vi "4AnInsADS1115.vi"() -> ()   [LabVIEW 2024]
uses:
  Controls/ConfigData.ctl
  Controls/ADS1115Mode.ctl
  Controls/ADS1115Mux.ctl
  Controls/ADS1115DataRate.ctl
  Controls/ADS1115PGA.ctl
  Driver/CTIPicoVISA.lvlib
panel:
  in  "Numeric":u16
  out "Data 2":string
  out "string":string
  out "Data":string
  in  "Configure ADS1115":T1={"Mode"=enum."Single-Shot", "MUX"=enum."Single AI3 - GND", "Data Rate"=enum."8 SPS", "PGA"=enum."FS = ±6.144V"}
  out "Waveform Chart":dbl(graph)
  out "loop":i32
  out "Identity":T6
  in  "Grove Connector":enum16{"I2C0", "I2C1"}(ring)
  in  "stop":bool
  in  "VISA resource name in":refnum<visa-resource-name>="COM14"
  out "error out":errorcluster
  # "https://wiki.seeedstudio.com/Grove-16-bit-ADC-ADS1115/"
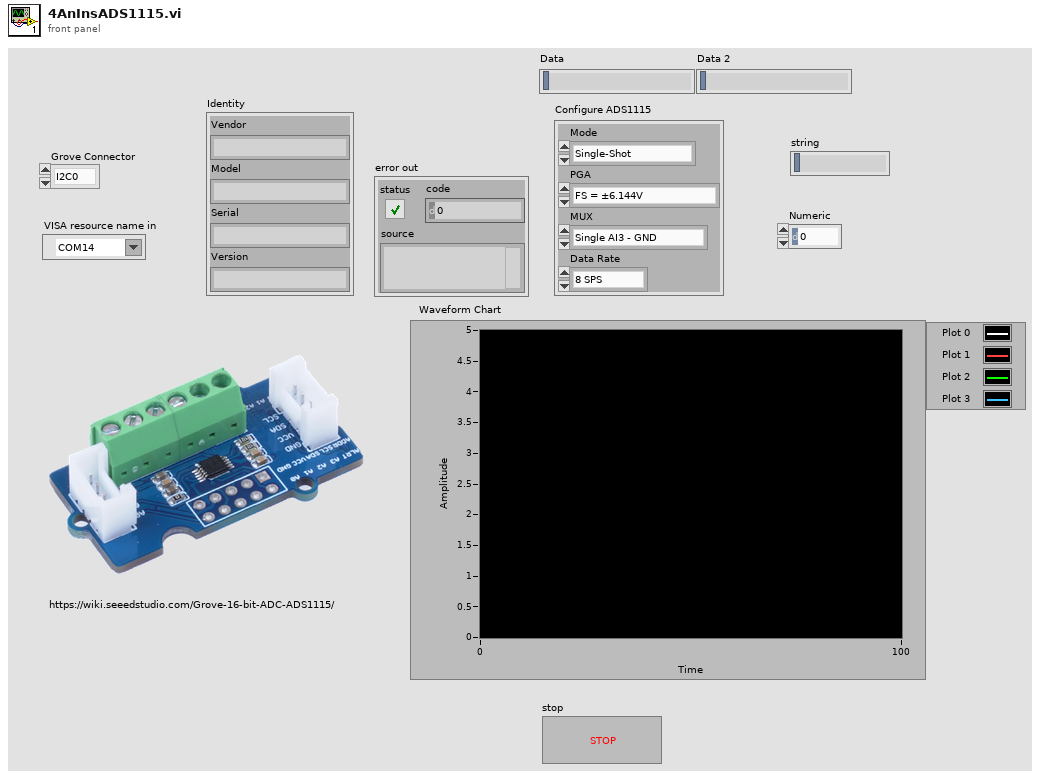
[diagram p1: front panel]
types:
  T1 = typedef "ConfigData.ctl" = cluster{"Mode":T2, "MUX":T3, "Data Rate":T4, "PGA":T5}
  T2 = typedef "ADS1115Mode.ctl" = enum16{"Continuous", "Single-Shot"}
  T3 = typedef "ADS1115Mux.ctl" = enum16{"Single AI0 - GND", "Single AI1 - GND", "Single AI2 - GND", "Single AI3 - GND"}
  T4 = typedef "ADS1115DataRate.ctl" = enum16{"8 SPS", "16 SPS", "32 SPS", "64 SPS", "128 SPS", "250 SPS", "475 SPS", "860 SPS"}
  T5 = typedef "ADS1115PGA.ctl" = enum16{"FS = ±6.144V", "FS = ±4.096V", "FS = ±2.048V", "FS = ±1.024V", "FS = ±0.512V", "FS = ±0.256V"}
  T6 = cluster{"Vendor":string, "Model":string, "Serial":string, "Version":string}
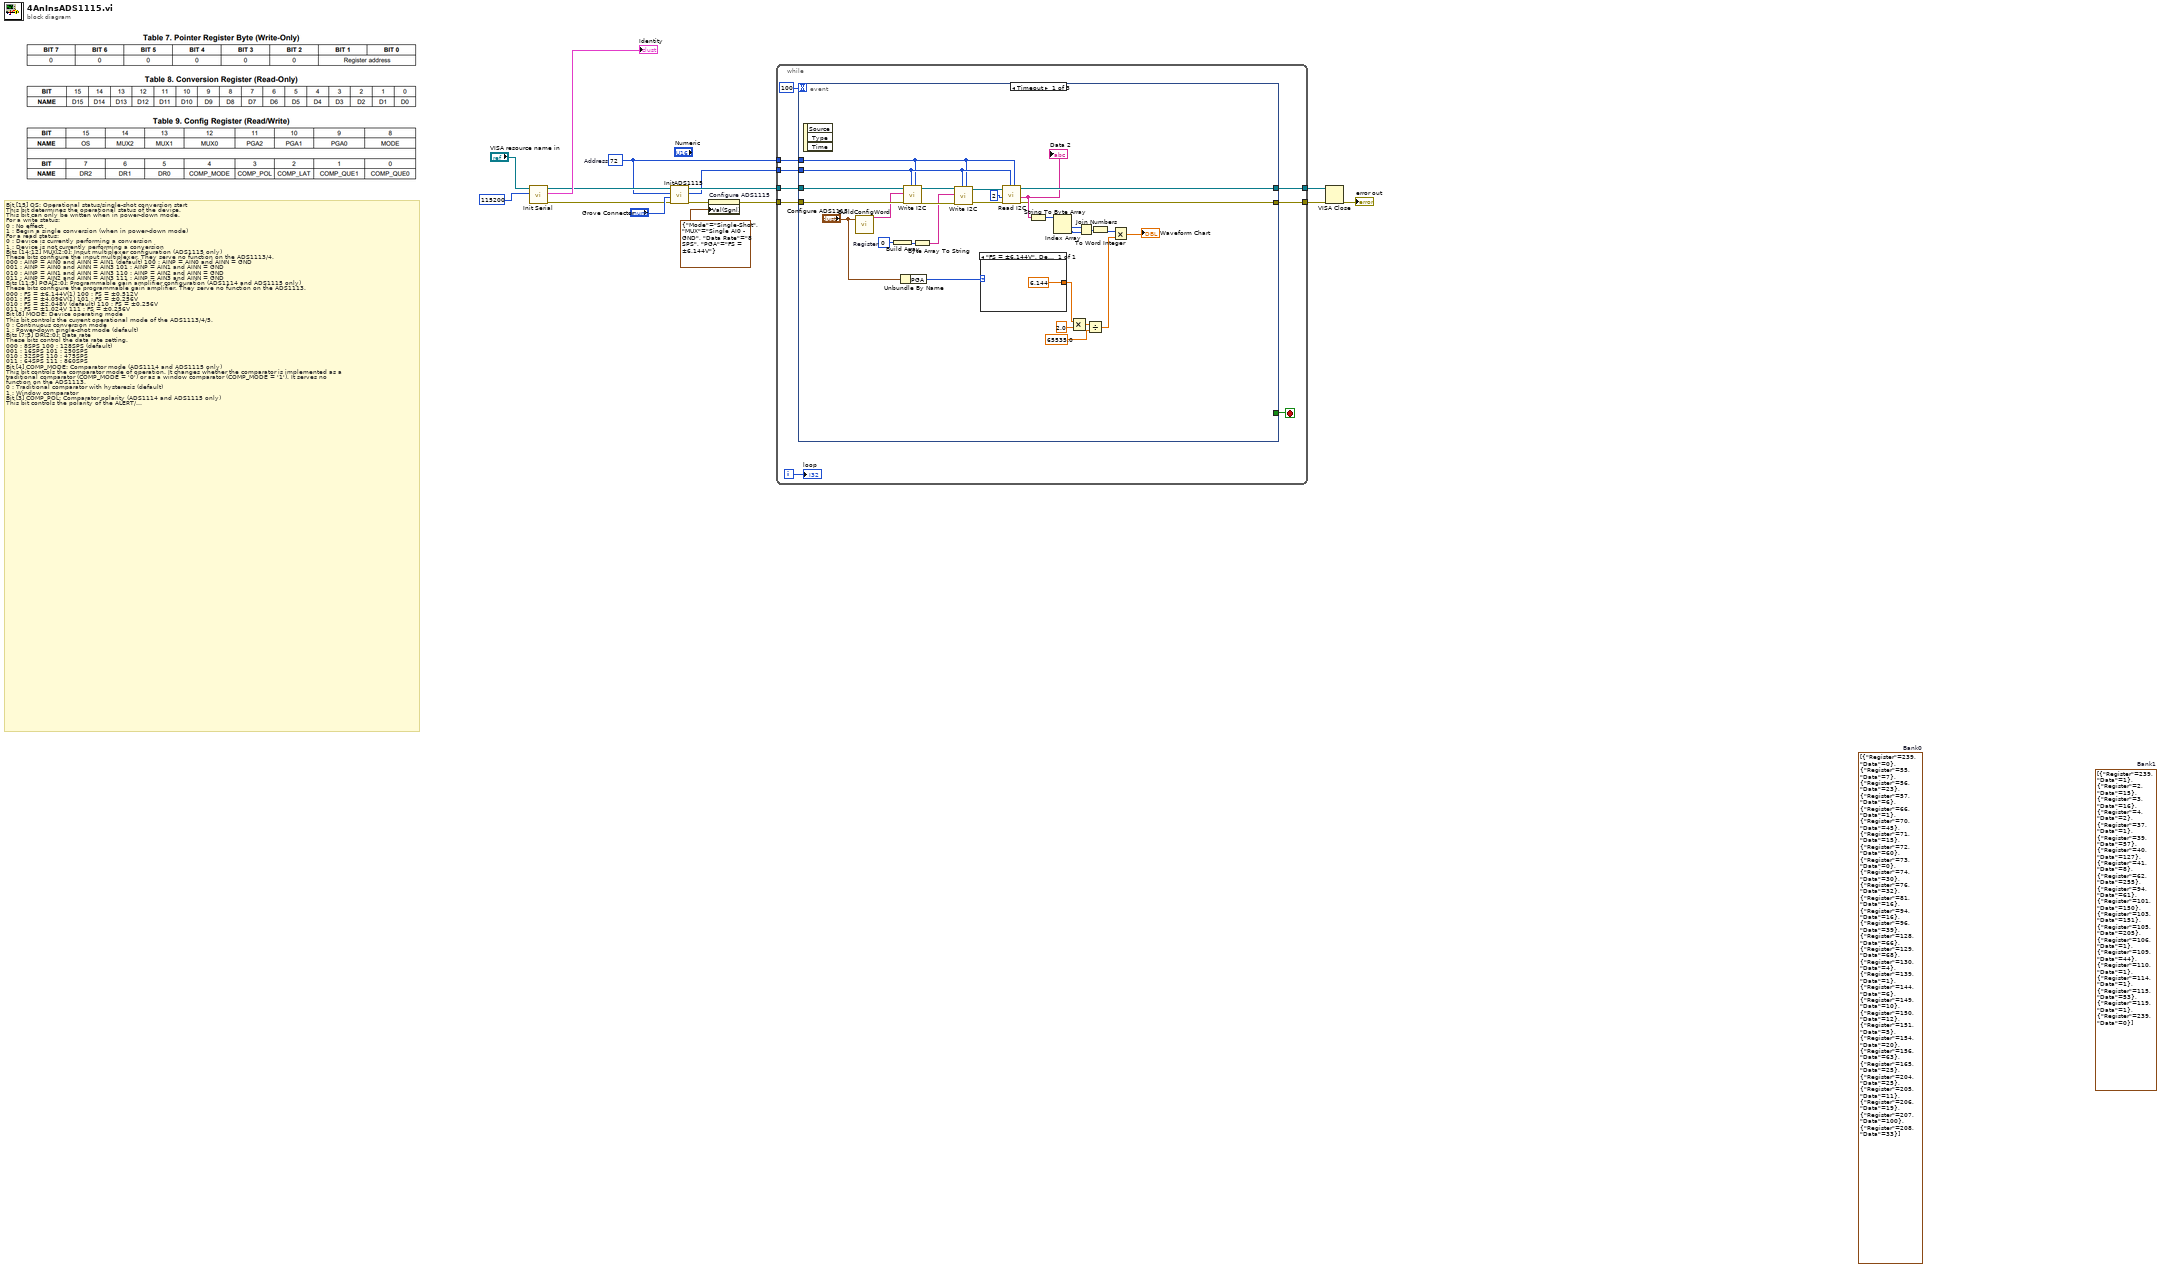
[diagram p0: block diagram]
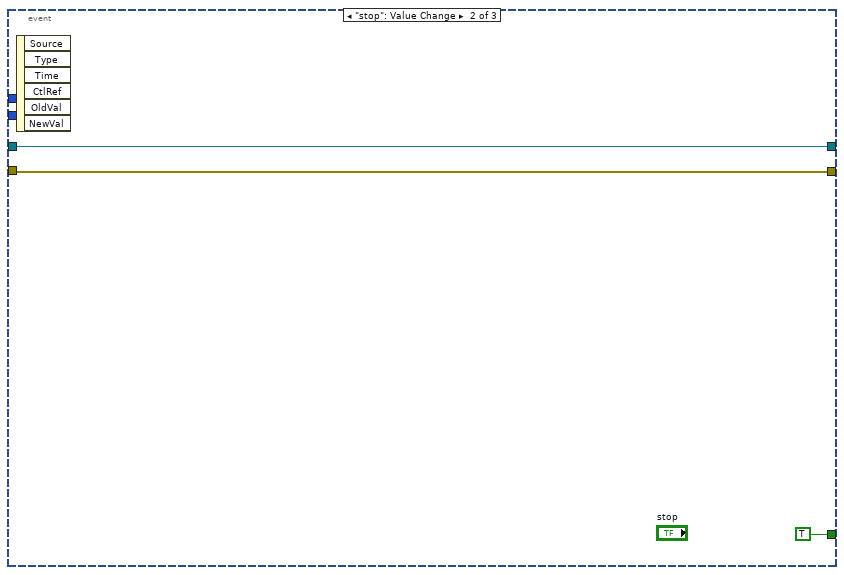
[diagram p2: hidden frame]
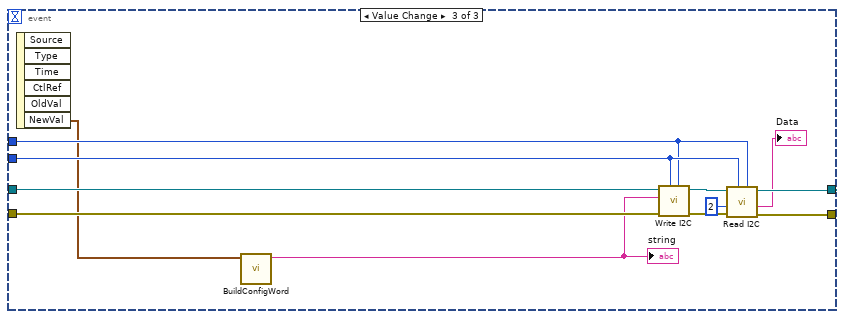
[diagram p3: hidden frame]
diagram:
  (unwired) cluster{"Register":u8, "Data":u8}[] [{"Register"=239, "Data"=0}, {"Register"=55, "Data"=7}, {"Register"=56, "Data"=23}, {"Register"=57, "Data"=6}, {"Register"=66, "Data"=1}, {"Register"=70, "Data"=45}, {"Register"=71, "Data"=15}, {"Register"=72, "Data"=60}, {"Register"=73, "Data"=0}, {"Register"=74, "Data"=30}, {"Register"=76, "Data"=32}, {"Register"=81, "Data"=16}, {"Register"=94, "Data"=16}, {"Register"=96, "Data"=39}, {"Register"=128, "Data"=66}, {"Register"=129, "Data"=68}, {"Register"=130, "Data"=4}, {"Register"=139, "Data"=1}, {"Register"=144, "Data"=6}, {"Register"=149, "Data"=10}, {"Register"=150, "Data"=12}, {"Register"=151, "Data"=5}, {"Register"=154, "Data"=20}, {"Register"=156, "Data"=63}, {"Register"=165, "Data"=25}, {"Register"=204, "Data"=25}, {"Register"=205, "Data"=11}, {"Register"=206, "Data"=19}, {"Register"=207, "Data"=100}, {"Register"=208, "Data"=33}]  # Bank0
  (unwired) cluster{"Register":u8, "Data":u8}[] [{"Register"=239, "Data"=1}, {"Register"=2, "Data"=15}, {"Register"=3, "Data"=16}, {"Register"=4, "Data"=2}, {"Register"=37, "Data"=1}, {"Register"=39, "Data"=57}, {"Register"=40, "Data"=127}, {"Register"=41, "Data"=8}, {"Register"=62, "Data"=255}, {"Register"=94, "Data"=61}, {"Register"=101, "Data"=150}, {"Register"=103, "Data"=151}, {"Register"=105, "Data"=205}, {"Register"=106, "Data"=1}, {"Register"=109, "Data"=44}, {"Register"=110, "Data"=1}, {"Register"=114, "Data"=1}, {"Register"=115, "Data"=53}, {"Register"=119, "Data"=1}, {"Register"=239, "Data"=0}]  # Bank1
  w4 = u8 72  # Address
  # "Bit [15] OS: Operational status/single-shot conversion start\nThis bit determines the operational status of the device.\nThis bit can only be written when in power-down mode.\nFor a write status:\n0 : No effect\n1 : Begin a single conversion (when in power-down mode)\nFor a read status:\n0 : Device is currently performing a conversion\n1 : Device is not currently performing a conversion\nBits [14:12] MUX[2:0]: Input multiplexer configuration (ADS1115 only)\nThese bits configure the input multiplexer. They serve no function on the ADS1113/4.\n000 : AINP = AIN0 and AINN = AIN1 (default) 100 : AINP = AIN0 and AINN = GND\n001 : AINP = AIN0 and AINN = AIN3 101 : AINP = AIN1 and AINN = GND\n010 : AINP = AIN1 and AINN = AIN3 110 : AINP = AIN2 and AINN = GND\n011 : AINP = AIN2 and AINN = AIN3 111 : AINP = AIN3 and AINN = GND\nBits [11:9] PGA[2:0]: Programmable gain amplifier configuration (ADS1114 and ADS1115 only)\nThese bits configure the programmable gain amplifier. They serve no function on the ADS1113.\n000 : FS = ±6.144V(1) 100 : FS = ±0.512V\n001 : FS = ±4.096V(1) 101 : FS = ±0.256V\n010 : FS = ±2.048V (default) 110 : FS = ±0.256V\n011 : FS = ±1.024V 111 : FS = ±0.256V\nBit [8] MODE: Device operating mode\nThis bit controls the current operational mode of the ADS1113/4/5.\n0 : Continuous conversion mode\n1 : Power-down single-shot mode (default)\nBits [7:5] DR[2:0]: Data rate\nThese bits control the data rate setting.\n000 : 8SPS 100 : 128SPS (default)\n001 : 16SPS 101 : 250SPS\n010 : 32SPS 110 : 475SPS\n011 : 64SPS 111 : 860SPS\nBit [4] COMP_MODE: Comparator mode (ADS1114 and ADS1115 only)\nThis bit controls the comparator mode of operation. It changes whether the comparator is implemented as a\ntraditional comparator (COMP_MODE = '0') or as a window comparator (COMP_MODE = '1'). It serves no\nfunction on the ADS1113.\n0 : Traditional comparator with hysteresis (default)\n1 : Window comparator\nBit [3] COMP_POL: Comparator polarity (ADS1114 and ADS1115 only)\nThis bit controls the polarity of the ALERT/RDY pin. When COMP_POL = '0' the comparator output is active\nlow. When COMP_POL='1' the ALERT/RDY pin is active high. It serves no function on the ADS1113.\n0 : Active low (default)\n1 : Active high\nBit [2] COMP_LAT: Latching comparator (ADS1114 and ADS1115 only)\nThis bit controls whether the ALERT/RDY pin latches once asserted or clears once conversions are within the\nmargin of the upper and lower threshold values. When COMP_LAT = '0', the ALERT/RDY pin does not latch\nwhen asserted. When COMP_LAT = '1', the asserted ALERT/RDY pin remains latched until conversion data\nare read by the master or an appropriate SMBus alert response is sent by the master, the device responds with\nits address, and it is the lowest address currently asserting the ALERT/RDY bus line. This bit serves no\nfunction on the ADS1113.\n0 : Non-latching comparator (default)\n1 : Latching comparator\nBits [1:0] COMP_QUE: Comparator queue and disable (ADS1114 and ADS1115 only)\nThese bits perform two functions. When set to '11', they disable the comparator function and put the\nALERT/RDY pin into a high state. When set to any other value, they control the number of successive\nconversions exceeding the upper or lower thresholds required before asserting the ALERT/RDY pin. They\nserve no function on the ADS1113.\n00 : Assert after one conversion\n01 : Assert after two conversions\n10 : Assert after four conversions\n11 : Disable comparator (default)\n(1) This parameter expresses the full-scale range of the ADC scaling. In no event should more than VDD + 0.3V be applied to this device."
  n1 = call "Init Serial.vi"("Baud (115200)"=u32 115200, "VISA resource name in"="VISA resource name in") -> ("error out"=w7:errorcluster, "Identity"=→"Identity":T6, "VISA resource name Out"=w8:refnum<visa-resource-name>)  [unwired: 7 in]
  n2 = call "InitADS1115.vi"("error in (no error)"=w7, "Grove Connector"="Grove Connector", "Address"=w4, "VISA Refnum in"=w8) -> ("error out"=w2:errorcluster, "Bus"=w5:u8, "VISA Refnum out"=w6:refnum<visa-resource-name>)  [unwired: 5 in]
  n3 = property on="Configure ADS1115" class="Clust (strict)"(error in=w2, "Val(Sgnl)"=T1 {"Mode"=enum."Single-Shot", "MUX"=enum."Single AI0 - GND", "Data Rate"=enum."8 SPS", "PGA"=enum."FS = ±6.144V"} ("Value (Signaling)")) -> (error out=w3:errorcluster)  [unwired: 1 in, 1 out]
  n4 = while {
    tunnel: w3 -> [w22]
    tunnel: [w18] -> w11
    tunnel: w6 -> [w23]
    tunnel: [w24] -> w10
    tunnel: w5 -> [w21]
    tunnel: w4 -> [w20]
    i -> [w19]
    stop <- w16 stop-if-true
    n5 = event shown="[0] Timeout" {
      selector: _ -> [_ _ _]
      dyn-events: _ -> [_ _ _]
      timeout: 100 -> [_ _ _]
      tunnel: [w53 w56 w67] -> w24
      tunnel: w23 -> [w45 w56 w63]
      tunnel: w22 -> [w44 w55 w66]
      tunnel: w21 -> [w38 _ w62]
      tunnel: w20 -> [w37 _ w61]
      tunnel: [w50 w55 w64] -> w18
      tunnel: [_ TRUE _] -> w16
      event Timeout {
        w35 = u8 0  # Register
        n6 = event-data() -> ()  [unwired: 1 in, 3 out]
        n7 = call "BuildConfigWord.vi"("NewVal"="Configure ADS1115") -> ("string"=w43:string)  [unwired: 10 in]
        n8 = Build Array(w35) -> (w36:u8[])
        n9 = Unbundle By Name("Configure ADS1115") -> ("PGA"=w32:T5)
        n10 = call "Write I2C.vi"("Address"=w37, "Bus"=w38, "error in (no error)"=w44, "Data"=w43, "VISA resource name in"=w45) -> ("error out"=w39:errorcluster, "VISA resource name"=w42:refnum<visa-resource-name>)  [unwired: 5 in]
        n11 = Byte Array To String(unsigned byte array=w36) -> (string=w34:string)
        n12 = call "Write I2C.vi"("Address"=w37, "Bus"=w38, "error in (no error)"=w39, "Data"=w34, "VISA resource name in"=w42) -> ("error out"=w40:errorcluster, "VISA resource name"=w41:refnum<visa-resource-name>)  [unwired: 5 in]
        n13 = case shown="\"FS = ±6.144V\", Default" w32 {
          tunnel: [6.144 ("Waveform Chart")] -> w27
          frame "FS = ±6.144V", Default {
          }
        }
        n14 = call "Read I2C.vi"("Address"=w37, "Bus"=w38, "error in (no error)"=w40, "Len"=u8 2, "VISA resource name in"=w41) -> ("error out"=w50:errorcluster, "Data"=w52:string, "VISA resource name"=w53:refnum<visa-resource-name>)  [unwired: 4 in]
        "Data 2" <- w52
        n15 = String To Byte Array(string=w52) -> (unsigned byte array=w49:u8[])
        n16 = Index Array(array=w49) -> (element #1=w48:u8, element #2=w47:u8)  [unwired: 2 in]
        n17 = Multiply(x=w27, y=2.0) -> (x*y=w29:dbl)
        n18 = Join Numbers(hi=w48, lo=w47) -> ((hi.lo)=w46:u16)
        n19 = Divide(x=w29, y=65535.0) -> (x/y=w26:dbl)
        n20 = To Word Integer(number=w46) -> (16bit integer=w31:i16)
        n21 = Multiply(x=w31, y=w26) -> (x*y=→"Waveform Chart":dbl)
      }
      event "stop": Value Change {
        n22 = event-data() -> ()  [unwired: 1 in, 6 out]
      }
      event Value Change {
        n23 = event-data() -> ("NewVal"=w59:T1)  [unwired: 1 in, 5 out]
        n24 = call "BuildConfigWord.vi"("NewVal"=w59) -> ("string"=w58:string)  [unwired: 10 in]
        "string" <- w58
        n25 = call "Write I2C.vi"("Address"=w61, "Bus"=w62, "error in (no error)"=w66, "Data"=w58, "VISA resource name in"=w63) -> ("error out"=w65:errorcluster, "VISA resource name"=w69:refnum<visa-resource-name>)  [unwired: 5 in]
        n26 = call "Read I2C.vi"("Address"=w61, "Bus"=w62, "error in (no error)"=w65, "Len"=u8 2, "VISA resource name in"=w69) -> ("error out"=w64:errorcluster, "Data"=→"Data":string, "VISA resource name"=w67:refnum<visa-resource-name>)  [unwired: 4 in]
      }
    }
    "loop" <- w19
  }
  n27 = VISA Close(VISA resource name=w10, error in (no error)=w11) -> (error out=→"error out":errorcluster)
